vi "auto_website.vi"   [LabVIEW 2023]
uses:
  <vilib>/Utility/file.llb/Read Delimited Spreadsheet (string).vi
types:
  T1 = enum16{"open", "replace", "create", "open or create", "replace or create", "replace or create with confirmation"}
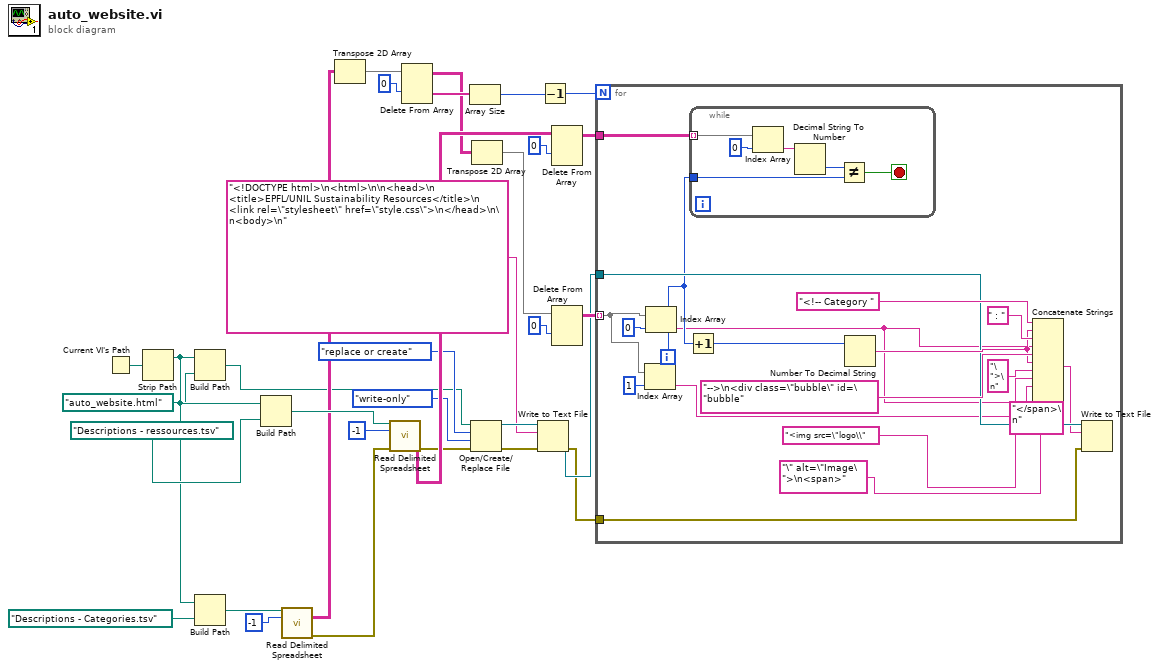
[diagram p0: block diagram]
diagram:
  n1 = Current VI's Path() -> (path=w26:path)
  n2 = Strip Path(path=w26) -> (stripped path=w17:path)  [unwired: 1 out]
  n3 = Build Path(base path=w17, name or relative path=path "auto_website.html") -> (appended path=w13:path)
  n4 = Build Path(base path=w17, name or relative path=path "Descriptions - Categories.tsv" ("Categories csv")) -> (appended path=w27:path)
  n5 = Build Path(base path=w17, name or relative path=path "Descriptions - ressources.tsv" ("Ressources csv")) -> (appended path=w29:path)
  n6 = call-poly <vilib>:"Read Delimited Spreadsheet.vi"("file path (dialog if empty)"=w27, "number of rows (all:-1)"=-1) -> ("all rows"=w23:string[][], "error out"=w12:errorcluster)  [unwired: 8 in, 4 out]
  n7 = Transpose 2D Array(2D array=w23) -> (transposed array=w21:string[][])
  n8 = call-poly <vilib>:"Read Delimited Spreadsheet.vi"("file path (dialog if empty)"=w29, "number of rows (all:-1)"=-1, "error in (no error)"=w12) -> ("all rows"=w25:string[][], "error out"=w11:errorcluster)  [unwired: 7 in, 4 out]
  n9 = Delete From Array(array=w21, index (row)=0) -> (deleted portion=w20:string[], array with subset deleted=w6:string[][])  [unwired: 2 in]
  n10 = Array Size(array=w20) -> (size(s)=w19:i32)
  n11 = Open/Create/Replace File(file path (use dialog)=w13, error in=w11, operation (0:open)=T1."replace or create", access (0:read/write)=enum16{"read/write", "read-only", "write-only"}."write-only") -> (refnum out=w10:refnum<file>, error out=w9:errorcluster)  [unwired: 2 in, 1 out]
  n12 = Transpose 2D Array(2D array=w6) -> (transposed array=w4:string[][])
  n13 = Write to Text File(file (use dialog)=w10, text="<!DOCTYPE html>\n<html>\n\n<head>\n    <title>EPFL/UNIL Sustainability Resources</title>\n    <link rel=\"stylesheet\" href=\"style.css\">\n</head>\n\n<body>\n", error in=w9) -> (refnum out=w2:refnum<file>, error out=w1:errorcluster)  [unwired: 1 in, 1 out]
  n14 = Decrement(x=w19) -> (x-1=w7:i32)
  n15 = Delete From Array(array=w25, index (row)=0) -> (array with subset deleted=w18:string[][])  [unwired: 2 in, 1 out]
  n16 = Delete From Array(array=w4, index (row)=0) -> (array with subset deleted=w3:string[][])  [unwired: 2 in, 1 out]
  n17 = for {
    N: w7 -> [_]
    tunnel: w18 -> [w51]
    tunnel: w3 -> [w37] mode=indexing
    tunnel: w2 -> [w43]
    tunnel: w1 -> [w42]
    i -> [w40]
    n18 = Index Array(array=w37, index=1) -> (element=w36:string)
    n19 = Index Array(array=w37, index=0) -> (element=w34:string)
    n20 = Increment(x=w40) -> (x+1=w39:i32)
    n21 = while {
      tunnel: w51 -> [w57] mode=indexing
      tunnel: w40 -> [w53]
      stop <- w52 stop-if-true
      n22 = Index Array(array=w57, index=0) -> (element=w55:string)
      n23 = Decimal String To Number(string=w55) -> (number=w54:i32)  [unwired: 2 in, 1 out]
      n24 = Not Equal?(x=w54, y=w53) -> (x != y?=w52:bool)
    }
    n25 = Number To Decimal String(number=w39) -> (decimal integer string=w46:string)  [unwired: 1 in]
    n26 = Concatenate Strings("<!-- Category " ("string"), w46, " : " ("string"), w34, "-->\n<div class=\"bubble\" id=\"bubble" ("string"), w46, "\">\n" ("string"), "<img src=\"logo\\" ("string"), w36, "\" alt=\"Image\">\n<span>" ("string"), w34, "</span>\n" ("string")) -> (w41:string)
    n27 = Write to Text File(file (use dialog)=w43, text=w41, error in=w42) -> ()  [unwired: 1 in, 3 out]
  }
